vi "Open.vi"(8 "error in":errorcluster, 9 "parameters":variant, 10 "file path":path, 11 "cRIO repo in":refnum<class "database file.lvclass">) -> (0 "error out":errorcluster, 2 "invalid?":bool, 3 "cRIO repo out":refnum<class "database file.lvclass">)   [LabVIEW 2013, in "database file.lvclass"]
doc: "Here we are specifying to read the configuration from a gXML file. And version management"
uses:
  database file.lvclass
  J1939 Library/Configuration/TypeDefs/J1939 db.ctl
  J1939 Library/Configuration/TypeDefs/J1939 db frame.ctl
  J1939 Library/Configuration/TypeDefs/J1939 db signal.ctl
  database file.lvclass/database file.ctl
  J1939 Library/J1939.lvlib
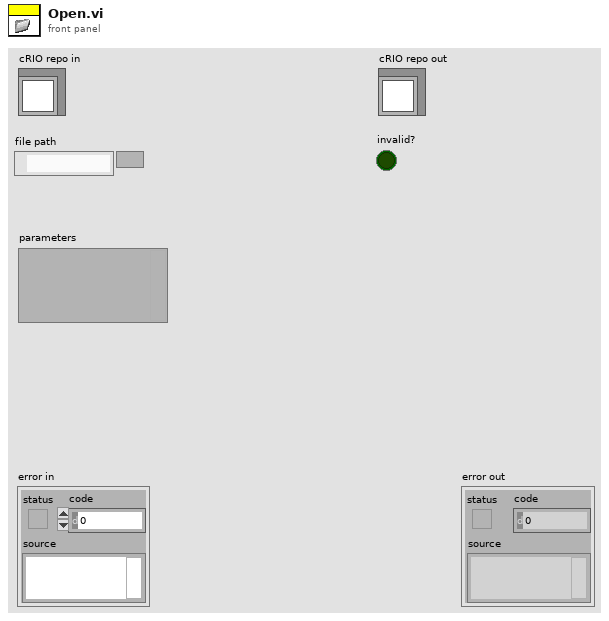
[diagram p1: front panel]
types:
  T1 = typedef "J1939.lvlib/J1939 db.ctl" = cluster{"BaudRate":u32, "CAN.IoMode":u32, "J1939 Network Address":u8, "Name":u64, "frames":T2[]}
  T2 = typedef "J1939.lvlib/J1939 db frame.ctl" = cluster{"name":string, "Priority":u8, "PGN":u32, "Reserved Bit":u8, "Data page":u8, "PDU Format":u8, "PDU Specific":u8, "Source Address":u8, "PayldLen":u32, "signals":T3[], "Comment":string, "can timing type":u32, "transmit time":dbl, "direction":u16}
  T3 = typedef "J1939.lvlib/J1939 db signal.ctl" = cluster{"NameShort":string, "SPN":i32, "StartBit":u32, "NumBits":u32, "DataType":u32, "ByteOrdr":u32, "ScaleFac":dbl, "ScaleOff":dbl, "Max":dbl, "Min":dbl, "Default":dbl, "Unit":string, "Comment":string}
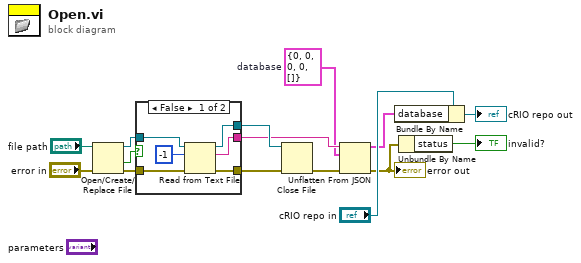
[diagram p0: block diagram]
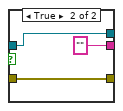
[diagram p2: hidden frame]
diagram:
  w4 = T1 {"BaudRate"=0, "CAN.IoMode"=0, "J1939 Network Address"=0, "Name"=0, "frames"=[]}  # database
  n1 = Open/Create/Replace File(file path (use dialog)="file path", error in="error in") -> (refnum out=w12:refnum<file>, cancelled=w13:bool, error out=w9:errorcluster)  [unwired: 4 in]
  n2 = case shown="False" w13 {
    tunnel: w12 -> [w21 w24]
    tunnel: [w20 w24] -> w11
    tunnel: [w19 w23] -> w10
    tunnel: w9 -> [w18 w23]
    tunnel: [w17 ""] -> w5
    frame False {
      n3 = Read from Text File(file (use dialog)=w21, count=-1, error in=w18) -> (refnum out=w20:refnum<file>, text=w17:string, error out=w19:errorcluster)  [unwired: 1 in, 1 out]
    }
    frame True {
    }
  }
  n4 = Close File(refnum=w11, error in=w10) -> (error out=w6:errorcluster)  [unwired: 1 out]
  n5 = Unflatten From JSON(JSON string=w5, type and defaults=w4, error in (no error)=w6) -> (value=w3:T1, error out=w2:errorcluster)  [unwired: 4 in]
  "error out" <- w2
  n6 = Bundle By Name(cluster="cRIO repo in", "database"=w3) -> (→"cRIO repo out":refnum<class "database file.lvclass">)
  n7 = Unbundle By Name(w2) -> ("status"=→"invalid?":bool)
